vi "Initialize.vi"(8 "error in (no error)":errorcluster, 9 "transceiver settings":T1, 10 "Transfer Groups Configurations":T2[](array[typedef]) {"Transfers"."channel configurations"."buffer offset" format="%d bytes"}, 11 "Transceiver in":refnum<class "Transceiver.lvclass">) -> (0 "error out":errorcluster, 3 "Transceiver out":refnum<class "Transceiver.lvclass">)   [LabVIEW 2017, in "DSF Core.lvlib" / "Transceiver.lvclass"]
uses:
  Transceiver.lvclass
  Configuration/Public/Controls/DSF Engine Transfer Group Configuration.ctl
  Configuration/Public/Controls/DSF Direction.ctl
  Configuration/Public/Controls/DSF Timing Info.ctl
  Configuration/Public/Controls/DSF Engine Transfer Configuration.ctl
  Configuration/Public/Controls/DSF Byte Order.ctl
  Configuration/Public/Controls/DSF Engine Channel Configuration.ctl
  Configuration/Public/Controls/DSF Data Type.ctl
  Configuration/Public/Controls/DSF Settings Info.ctl
  DSF Core.lvlib
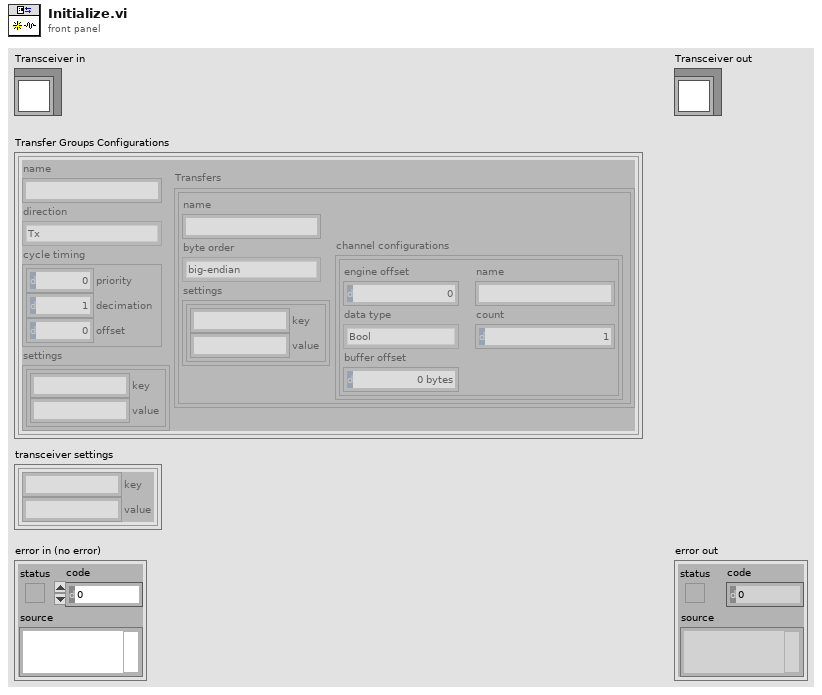
[diagram p1: front panel]
types:
  T1 = typedef "DSF Core.lvlib/DSF Settings Info.ctl" = cluster{"key":string, "value":string}[]
  T2 = typedef "DSF Core.lvlib/DSF Engine Transfer Group Configuration.ctl" = cluster{"name":string, "direction":T3, "cycle timing":T4, "Transfers":T5[], "settings":T1}
  T3 = typedef "DSF Core.lvlib/DSF Direction.ctl" = enum8{"Tx", "Rx"}
  T4 = typedef "DSF Core.lvlib/DSF Timing Info.ctl" = cluster{"priority":u64, "decimation":u64, "offset":u64}
  T5 = typedef "DSF Core.lvlib/DSF Engine Transfer Configuration.ctl" = cluster{"name":string, "byte order":T6, "channel configurations":T7[], "settings":T1}
  T6 = typedef "DSF Core.lvlib/DSF Byte Order.ctl" = enum8{"big-endian", "little-endian"}
  T7 = typedef "DSF Core.lvlib/DSF Engine Channel Configuration.ctl" = cluster{"engine offset":u64, "name":string, "data type":T8, "count":u64, "buffer offset":u64}
  T8 = typedef "DSF Core.lvlib/DSF Data Type.ctl" = enum8{"Bool", "SGL", "DBL", "I8", "I16", "I32", "I64", "U8", "U16", "U32", "U64"}
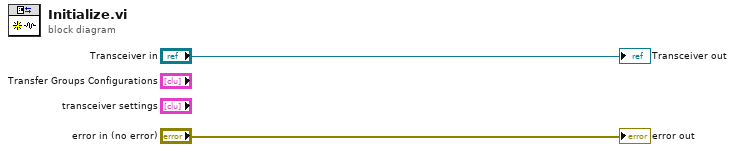
[diagram p0: block diagram]
diagram:
  "error out" <- "error in (no error)"
  "Transceiver out" <- "Transceiver in"
